vi "Cross_spectra.vi"(4 "block number":i32, 5 "S11 input array":dbl[](array[numeric]) format="%.2f", 6 "sampling frequency":dbl format="%.2f", 7 "S22 input array":dbl[](array[numeric]) format="%.2f", 8 "Im(S12) input array":dbl[](array[numeric]) format="%.2f", 9 "Re(S12) input array":dbl[](array[numeric]) format="%.2f", 10 "U2":dbl[](array[numeric]) format="%.2f", 11 "U1":dbl[](array[numeric]) format="%.2f") -> (0 "Im(S12) output array":dbl[](array[numeric]) format="%.2f", 1 "Re(S12) output array":dbl[](array[numeric]) format="%.2f", 2 "Phase array":dbl[](array[numeric]) format="%.2f", 3 "Coherence array":dbl[](array[numeric]) format="%.2f")   [LabVIEW 2011]
doc: "This VI produces ensemble-averaged Coherence and Phase information using a Cross-Power Spectrum. Inputs from the individual Power Spectra are required to scale the coherence array.\nNote that the DC element of the arrays is removed; output arrays commence at 1.dF, not 0Hz. The outputs are single sided."
uses:
  <vilib>/Analysis/2dsp.llb/Cross Power (DBL).vi
  <vilib>/Analysis/baseanly.llb/Mean.vi
  <vilib>/Analysis/NI_AALPro.lvlib
panel:
  out "error":i32
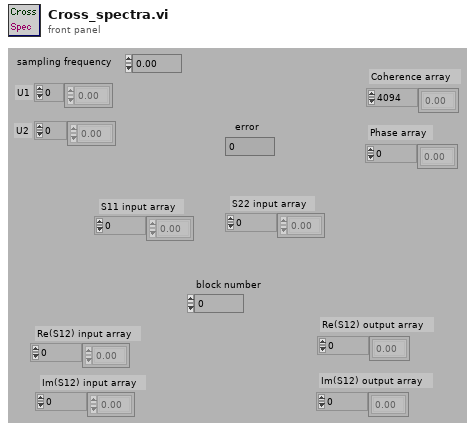
[diagram p1: front panel]
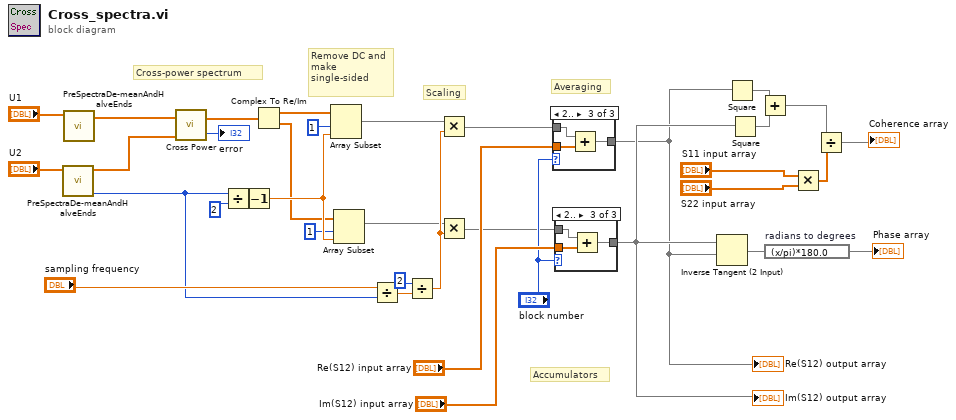
[diagram p0: block diagram]
diagram:
  # "Cross-power spectrum"
  # "Remove DC and make single-sided"
  # "Averaging"
  # "Scaling"
  # "Accumulators"
  n1 = call "PreSpectraDe-meanAndHalveEnds.vi"("Array"="U2") -> ("length"=w3:i32, "PreppedArray"=w5:dbl[])  [unwired: 9 in]
  n2 = call "PreSpectraDe-meanAndHalveEnds.vi"("Array"="U1") -> ("PreppedArray"=w7:dbl[])  [unwired: 9 in, 1 out]
  n3 = call-poly <vilib>:"Cross Power.vi"("Y"=w5, "X"=w7) -> ("error"=→"error":i32, "Sxy"=w23:cdb[])
  n4 = Divide(x=w3, y=2) -> (x/y=w29:dbl)
  n5 = Decrement(x=w29) -> (x-1=w28:dbl)
  n6 = Complex To Re/Im(x + iy=w23) -> (x=w22:dbl[], y=w21:dbl[])
  n7 = Array Subset(array=w22, index=1, length=w28) -> (w35:dbl[])
  n8 = Array Subset(array=w21, index=1, length=w28) -> (w25:dbl[])
  n9 = Divide(x="sampling frequency", y=w3) -> (x/y=w13:dbl)
  n10 = Divide(x=2, y=w13) -> (x/y=w26:dbl)
  n11 = Multiply(x=w35, y=w26) -> (x*y=w16:dbl[])
  n12 = Multiply(x=w25, y=w26) -> (x*y=w17:dbl[])
  n13 = case shown="2.." "block number" {
    tunnel: [w37 w38 w41] -> w10
    tunnel: w16 -> [w37 w38 w40]
    tunnel: "Re(S12) input array" -> [_ _ w39]
    frame ..0 {
    }
    frame 1 {
    }
    frame 2.. {
      n14 = Add(x=w40, y=w39) -> (x+y=w41:dbl[])
    }
  }
  "Re(S12) output array" <- w10
  n15 = case shown="2.." "block number" {
    tunnel: [w42 w43 w46] -> w11
    tunnel: w17 -> [w42 w43 w45]
    tunnel: "Im(S12) input array" -> [_ _ w44]
    frame ..0 {
    }
    frame 1 {
    }
    frame 2.. {
      n16 = Add(x=w45, y=w44) -> (x+y=w46:dbl[])
    }
  }
  "Im(S12) output array" <- w11
  n17 = Inverse Tangent (2 Input)(1:w10, 2:w11) -> (0:w2:dbl[])
  n18 = Square(x=w10) -> (x^2=w20:dbl[])
  n19 = Square(x=w11) -> (x^2=w19:dbl[])
  n20 = Add(x=w20, y=w19) -> (x+y=w18:dbl[])
  n21 = expression code="(x/pi)*180.0" "radians to degrees"(w2) -> (→"Phase array":dbl[])
  n22 = Multiply(x="S11 input array", y="S22 input array") -> (x*y=w31:dbl[])
  n23 = Divide(x=w18, y=w31) -> (x/y=→"Coherence array":dbl[])
